vi "AppConfig.vi"(8 "error in (no error)":errorcluster) -> (0 "error out":errorcluster, 3 "value":u32)   [LabVIEW 2019]
uses:
  <vilib>/Utility/config.llb/Read Key (U32).vi
  <vilib>/Utility/config.llb/NI_LVConfig.lvlib
  <vilib>/Utility/config.llb/Write Key (U32).vi
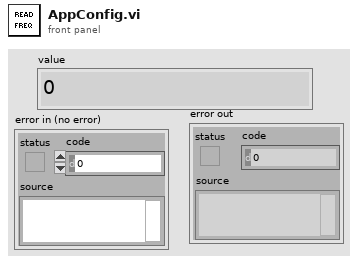
[diagram p1: front panel]
types:
  T1 = typedef "NI_LVConfig.lvlib/Config Data RefNum.ctl" = refnum<k1>
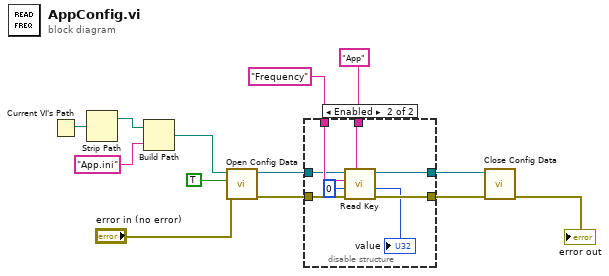
[diagram p0: block diagram]
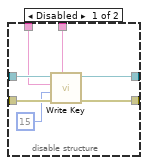
[diagram p2: hidden frame]
diagram:
  n1 = Current VI's Path() -> (path=w9:path)
  n2 = Strip Path(path=w9) -> (stripped path=w8:path)  [unwired: 1 out]
  n3 = Build Path(base path=w8, name or relative path="App.ini") -> (appended path=w6:path)
  n4 = call <vilib>:"Open Config Data.vi"("error in (no error)"="error in (no error)", "create file if necessary (T)"=TRUE, "configuration file path"=w6) -> ("error out"=w12:errorcluster, "refnum"=w13:T1)  [unwired: 6 in, 1 out]
  n5 = disable-structure shown="Enabled" {
    disable-tunnel: w13 -> [w20 w26]
    disable-tunnel: w12 -> [w19 w24]
    disable-tunnel: [w18 w22] -> w11
    disable-tunnel: [w17 w23] -> w10
    disable-tunnel: "App" ("section") -> [w16 w28]
    disable-tunnel: "Frequency" ("key") -> [w15 w27]
    frame Disabled {
      n6 = call-poly <vilib>:"Write Key.vi"("section"=w16, "error in (no error)"=w19, "value"=u32 15, "key"=w15, "refnum"=w20) -> ("error out"=w17:errorcluster, "refnum out"=w18:T1)  [unwired: 4 in, 1 out]
    }
    frame Enabled {
      n7 = call-poly <vilib>:"Read Key.vi"("section"=w28, "error in (no error)"=w24, "default value"=u32 0, "key"=w27, "refnum"=w26) -> ("error out"=w23:errorcluster, "value"=→"value":u32, "refnum out"=w22:T1)  [unwired: 3 in, 1 out]
    }
  }
  n8 = call <vilib>:"Close Config Data.vi"("error in (no error)"=w10, "refnum"=w11) -> ("error out"=→"error out":errorcluster)  [unwired: 8 in, 1 out]
